vi "Discover Nodes.vi"(8 "error in":errorcluster, 11 "Network Management in":refnum<class "Network Management.lvclass">) -> (0 "error out":errorcluster, 3 "Network Management out":refnum<class "Network Management.lvclass">)   [LabVIEW 2020, in "CANopen.lvlib" / "Network Management.lvlib" / "Network Management.lvclass"]
uses:
  Network Management.lvclass
  Network Management.lvclass/Network Management.ctl
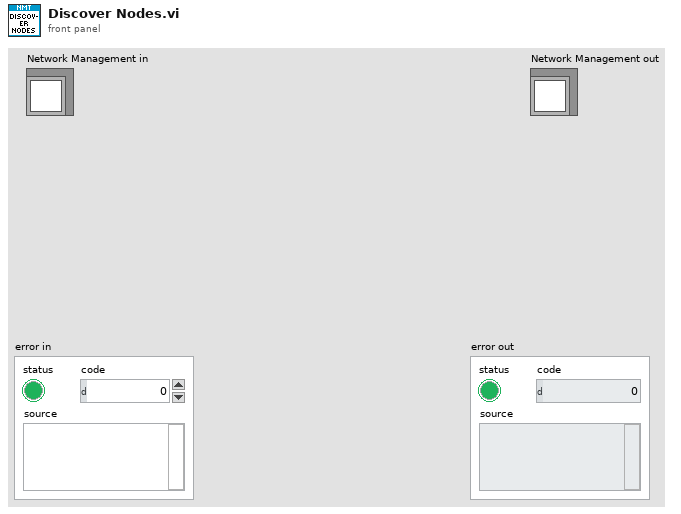
[diagram p1: front panel]
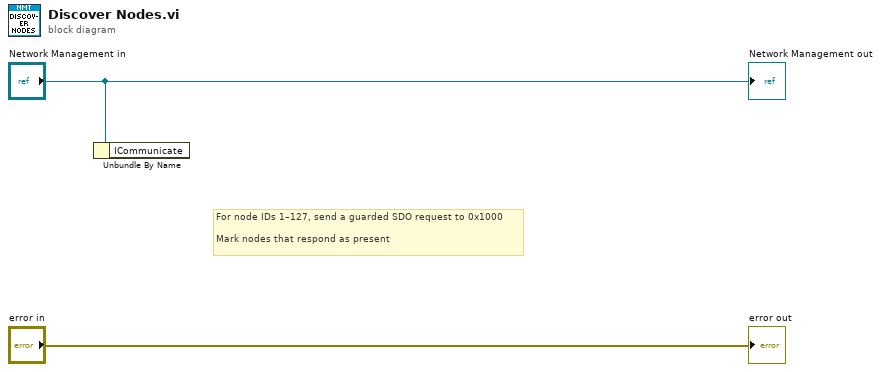
[diagram p0: block diagram]
diagram:
  # "For node IDs 1–127, send a guarded SDO request to 0x1000\n\nMark nodes that respond as present"
  n1 = Unbundle By Name("Network Management in") -> ()  [unwired: 1 out]
  "Network Management out" <- "Network Management in"
  "error out" <- "error in"
